vi "XGT 연속읽기.vi"(5 "데이터개수":string="02", 7 "변수이름":string="%MW000", 8 "error in (no error)":errorcluster caption="에러 입력(에러 없음)", 9 "변수길이":string="06", 10 "국번":string="0A", 11 "VISA 리소스 이름":refnum<visa-resource-name>) -> (0 "error out":errorcluster caption="에러 출력", 1 "배열":i32[](array[numeric]), 2 "버퍼 읽기 (응답)":string, 3 "VISA 리소스 이름 출력":refnum<visa-resource-name>, 4 "데이터":string, 6 "연속연결 Enquire문":string)   [LabVIEW 2012]
panel:
  out "에러 코드":string
  out "국번 2":string
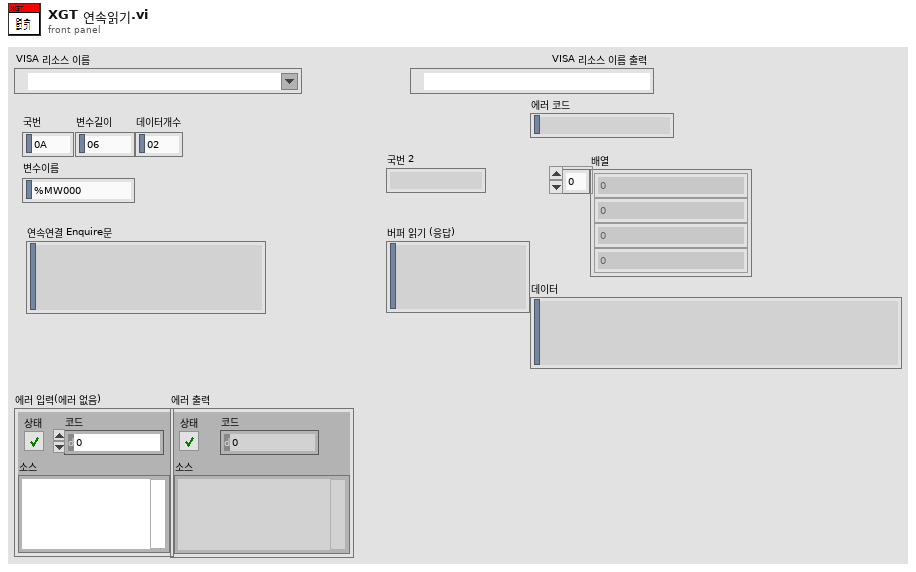
[diagram p1: front panel]
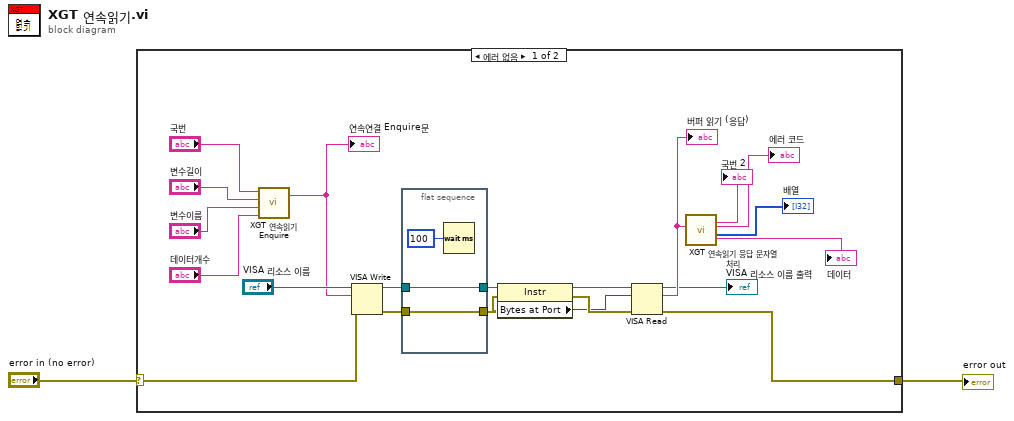
[diagram p0: block diagram]
diagram:
  n1 = case shown="에러 없음" "error in (no error)" {
    selector: "error in (no error)" -> [w20 w27]
    tunnel: [w5 w27] -> w1
    frame No Error {
      n2 = call "XGT 연속읽기 Enquire.vi"("데이터개수"="데이터개수", "변수이름"="변수이름", "변수길이"="변수길이", "국번"="국번") -> ("연속연결 Enquire문"=w13:string)  [unwired: 7 in]
      "연속연결 Enquire문" <- w13
      n3 = VISA Write(VISA resource name="VISA 리소스 이름", write buffer=w13, error in (no error)=w20) -> (VISA resource name out=w22:refnum<visa-resource-name>, error out=w23:errorcluster)  [unwired: 1 out]
      n4 = flat-sequence {
        tunnel: w23 -> [w26]
        tunnel: [w26] -> w17
        tunnel: w22 -> [w25]
        tunnel: [w25] -> w18
        frame #0 {
          n5 = Wait (ms)(milliseconds to wait=u32 100 ("대기 시간(ms)")) -> ()  [unwired: 1 out]
        }
      }
      n6 = property class="Instr"(reference=w18, error in=w17) -> (reference out=w16:refnum<visa-resource-name>, error out=w19:errorcluster, "Bytes at Port"=w15:u32)
      n7 = VISA Read(VISA resource name=w16, byte count=w15, error in (no error)=w19) -> (VISA resource name out=→"VISA 리소스 이름 출력":refnum<visa-resource-name>, read buffer=w14:string, error out=w5:errorcluster)  [unwired: 1 out]
      "버퍼 읽기 (응답)" <- w14
      n8 = call "XGT 연속읽기 응답 문자열 처리.vi"("응답"=w14) -> ("배열"=→"배열":i32[], "에러 코드"=→"에러 코드":string, "데이터"=→"데이터":string, "국번"=→"국번 2":string)  [unwired: 5 in, 2 out]
    }
    frame Error {
    }
  }
  "error out" <- w1
